vi "Configure Operation Mode.vi"(0 "VISA resource name":refnum<visa-resource-name>, 5 "Operation Mode (0:Program)":u16(ring) items=["Program", "Manual", "DC+", "DC-"], 11 "error in (no error)":errorcluster) -> (4 "VISA resource name out":refnum<visa-resource-name>, 15 "error out":errorcluster)   [LabVIEW 2016, in "APT 300XAC Series.lvlib"]
doc: "Sets the <B>Operation Mode</B> of the power source instrument.\n\nThe option places the AC power source into one of several modes (Program/Manual/DC+/DC-). In the program mode the operator will have the ability to program individual memories and steps with user selectable testing parameters such as test time, high and low limits, etc. \n\nIn the manual mode the operator will have limited choices in selecting and editing testing parameters. The key difference is that in manual mode the operator can not connect steps or have fixed testing times. The output is either on or off in the manual mode.\n\nIn the DC+/DC- mode the operator can select either a positive or negative DC output. This selection will only be available if the DC option has been installed on the AC power source."
uses:
  APT 300XAC Series.lvlib
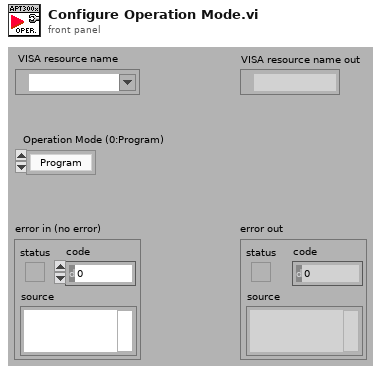
[diagram p1: front panel]
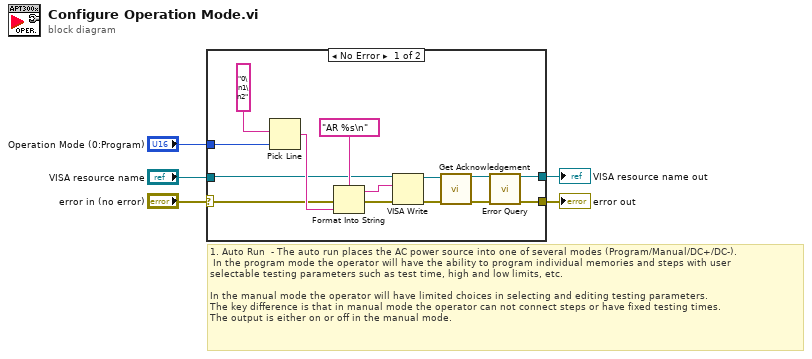
[diagram p0: block diagram]
diagram:
  # "1.\tAuto Run  - The auto run places the AC power source into one of several modes (Program/Manual/DC+/DC-).\n In the program mode the operator will have the ability to program individual memories and steps with user \nselectable testing parameters such as test time, high and low limits, etc.  \n\nIn the manual mode the operator will have limited choices in selecting and editing testing parameters.  \nThe key difference is that in manual mode the operator can not connect steps or have fixed testing times.  \nThe output is either on or off in the manual mode."
  n1 = case shown="No Error" "error in (no error)" {
    selector: "error in (no error)" -> [w6 w21]
    tunnel: "VISA resource name" -> [w7 w20]
    tunnel: [w14 w20] -> w4
    tunnel: [w13 w21] -> w3
    tunnel: "Operation Mode (0:Program)" -> [w19 _]
    frame No Error {
      n2 = Pick Line(multi-line string="0\n1\n2" ("Enum1"), line index=w19) -> (output string=w16:string)  [unwired: 1 in]
      n3 = Format Into String(format string="AR %s\n" ("Command"), error in=w6, w16) -> (resulting string=w17:string, error out=w12:errorcluster)  [unwired: 1 in]
      n4 = VISA Write(VISA resource name=w7, write buffer=w17, error in (no error)=w12) -> (VISA resource name out=w10:refnum<visa-resource-name>, error out=w9:errorcluster)  [unwired: 1 out]
      n5 = call "Get Acknowledgement.vi"("VISA resource name"=w10, "error in (no error)"=w9) -> ("VISA resource name out"=w11:refnum<visa-resource-name>, "error out"=w8:errorcluster)  [unwired: 12 in]
      n6 = call "Error Query.vi"("VISA resource name"=w11, "error in (no error)"=w8) -> ("VISA resource name out"=w14:refnum<visa-resource-name>, "error out"=w13:errorcluster)  [unwired: 10 in, 2 out]
    }
    frame Error {
    }
  }
  "error out" <- w3
  "VISA resource name out" <- w4
